vi "Init UserPwd DB Config Obj.vi"(8 "error in (no error)":errorcluster, 11 "VacuumLines Configuration in":refnum<class "VacuumLines Configuration.lvclass">) -> (0 "error out":errorcluster, 2 "UserPwd DB Configuration Obj":refnum<class "UserPwd DB Configuration.lvclass">, 3 "VacuumLines Configuration out":refnum<class "VacuumLines Configuration.lvclass">)   [LabVIEW 2016, in "Hardware.lvlib" / "VacuumLine.lvlib" / "VacuumLines Configuration.lvclass"]
uses:
  <userlib>/Common Components/Hardware/Abstract System/VacuumLine/VacuumLines Configuration/VacuumLines Configuration.lvclass
  C:/Program Files (x86)/National Instruments/LabVIEW 2016/user.lib/Configuration Dialog Actor/Configuration.lvclass
  <userlib>/Common Components/UserPwd DB/UserPwd DB Config/UserPwd DB Configuration.lvclass
  <userlib>/Common Components/UserPwd DB/UserPwd DB Config/UserPwd DB Configuration.lvclass/UserPwd DB Configuration.ctl
  <userlib>/Common Components/Hardware/Abstract System/VacuumLine/VacuumLines Configuration/VacuumLines Configuration.lvclass/VacuumLines Configuration.ctl
  <userlib>/Configuration Dialog Actor/Configuration.lvclass/Configuration.ctl
  <userlib>/Common Components/Hardware/Abstract System/VacuumLine/VacuumLines Configuration/Accessors/Read VacuumLines Obj.vi
  <userlib>/Configuration Dialog Actor/Accessors/Read Change Display.vi
  <userlib>/Configuration Dialog Actor/Accessors/Read Sub Panel.vi
  <userlib>/Configuration Dialog Actor/Accessors/Read Title.vi
  <userlib>/Configuration Dialog Actor/Accessors/Read Categories.vi
  <userlib>/Configuration Dialog Actor/Accessors/Write Change Display.vi
  <userlib>/Configuration Dialog Actor/Accessors/Write Sub Panel.vi
  <userlib>/Configuration Dialog Actor/Accessors/Write Title.vi
  <userlib>/Configuration Dialog Actor/Accessors/Write Categories.vi
  <userlib>/Common Components/Hardware/Abstract System/VacuumLine/VacuumLines/VacuumLines.lvclass
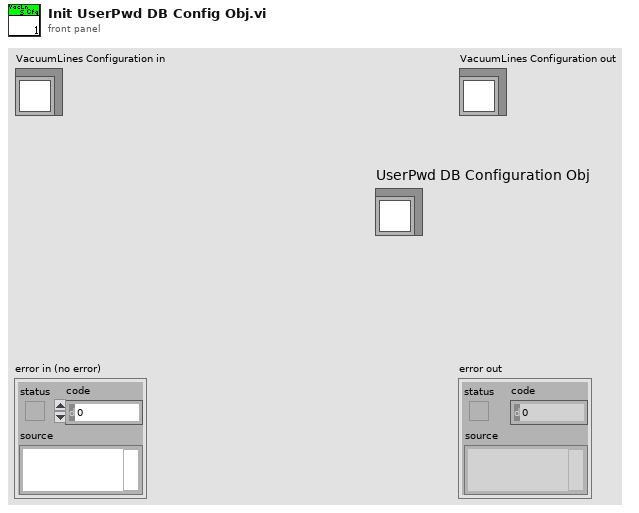
[diagram p1: front panel]
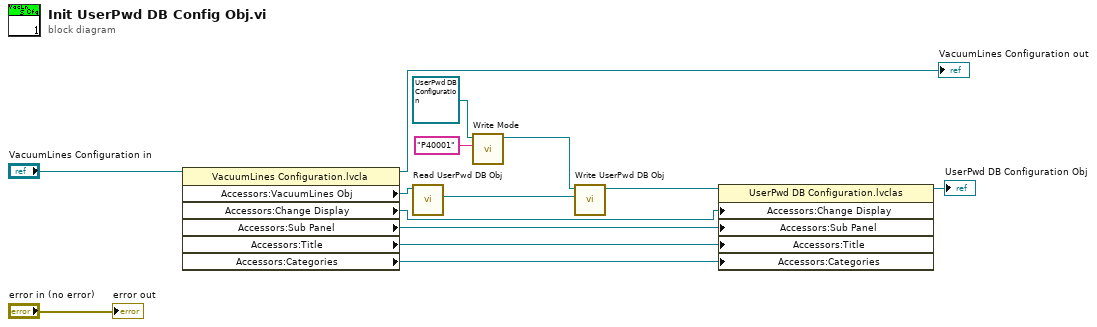
[diagram p0: block diagram]
diagram:
  n1 = property class="VacuumLines Configuration.lvcla"(reference="VacuumLines Configuration in") -> (reference out=→"VacuumLines Configuration out":refnum<class "VacuumLines Configuration.lvclass">, "Accessors:VacuumLines Obj"=w11:refnum<class "VacuumLines.lvclass">, "Accessors:Change Display"=w10:refnum<user-event>, "Accessors:Sub Panel"=w9:refnum<vi>, "Accessors:Title"=w8:refnum<vi>, "Accessors:Categories"=w7:refnum<vi>)  [unwired: 1 in, 1 out]
  n2 = call <userlib>:"Read UserPwd DB Obj.vi"("VacuumLines in"=w11) -> ("UserPwd DB.lvlib:UserPwd DB.lvclass"=w4:refnum<class "UserPwd DB.lvclass">)  [unwired: 9 in, 1 out]
  n3 = call <userlib>:"Write Mode.vi"("Mode"="P40001", "UserPwd DB Configuration in"=refnum<class "UserPwd DB Configuration.lvclass"> refnum ("UserPwd DB.lvlib:UserPwd DB Configuration.lvclass")) -> ("UserPwd DB Configuration out"=w2:refnum<class "UserPwd DB Configuration.lvclass">)  [unwired: 9 in]
  n4 = call <userlib>:"Write UserPwd DB Obj.vi"("UserPwd DB.lvlib:UserPwd DB.lvclass"=w4, "UserPwd DB Configuration in"=w2) -> ("UserPwd DB Configuration out"=w3:refnum<class "UserPwd DB Configuration.lvclass">)  [unwired: 9 in]
  n5 = property class="UserPwd DB Configuration.lvclas"(reference=w3, "Accessors:Change Display"=w10, "Accessors:Sub Panel"=w9, "Accessors:Title"=w8, "Accessors:Categories"=w7) -> (reference out=→"UserPwd DB Configuration Obj":refnum<class "UserPwd DB Configuration.lvclass">)  [unwired: 1 in, 1 out]
  "error out" <- "error in (no error)"
